vi "Receive.vi"(11 "Base Queue in":refnum<class "Base Queue.lvclass">) -> (2 "Msg Strategy":refnum<class "Msg Strategy.lvclass">, 3 "Base Queue out":refnum<class "Base Queue.lvclass">)   [LabVIEW 2021, in "jettl.lvlib" / "Base Queue.lvlib" / "Base Queue.lvclass"]
uses:
  Base Queue.lvclass
  Msg Strategy/Msg Strategy.lvclass
  Base Queue.lvclass/Base Queue.ctl
  Self Queue/Self Queue.lvlib
  Merge Error Msg Strategy/Merge Error Msg Strategy.lvlib
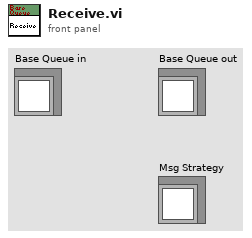
[diagram p1: front panel]
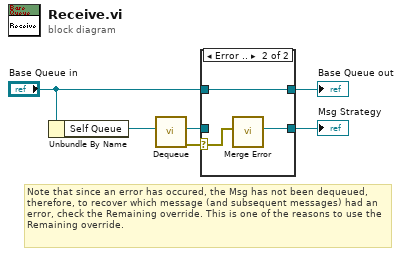
[diagram p0: block diagram]
diagram:
  # "Note that since an error has occured, the Msg has not been dequeued, therefore, to recover which message (and subsequent messages) had an error, check the Remaining override. This is one of the reasons to use the Remaining override."
  n1 = Unbundle By Name("Base Queue in") -> ("Self Queue"=w3:refnum<data-value>)
  n2 = call "Dequeue.vi"("Self Queue"=w3) -> ("error out"=w2:errorcluster, "Msg Strategy"=w1:refnum<class "Msg Strategy.lvclass">)  [unwired: 9 in]
  n3 = case shown="Error .." w2 {
    selector: w2 -> [_ w10]
    tunnel: w1 -> [w7 _]
    tunnel: "Base Queue in" -> [w8 w9]
    tunnel: [w8 w9] -> w6
    tunnel: [w7 w11] -> w5
    frame No Error {
    }
    frame Error {
      n4 = call "Merge Error.vi"("Error"=w10) -> ("Msg Strategy"=w11:refnum<class "Msg Strategy.lvclass">)  [unwired: 10 in]
    }
  }
  "Base Queue out" <- w6
  "Msg Strategy" <- w5
